vi "MultiCamExample.vi"() -> ()   [LabVIEW 2015]
panel:
  out "Numeric":i32
  out "Initialize Done":bool
  out "time":u32
  in  "Enabled/Disabled 1":bool
  in  "Load Picture 1":bool
  in  "Script Index 1":i32=1
  out "data string 1":string="1113.00\r\n935.00\r\n"
  out "VarName 1":string="up_ROI0_PM_Position_x\r\nup_ROI0_PM_Position_y\r\n"
  in  "Cam Index 1":i32=1
  in  "coordinate space 1":bool
  out "VarName 0":string="up_ROI0_PM_Position_x\r\nup_ROI0_PM_Position_y\r\n"
  in  "Script Index 0":i32
  in  "CameraName":string[](array[string])=["cam0"]
  in  "Load File Path":string[](array[string])=["C:\\Code\\Washers.png"]
  in  "script path":string[](array[string])=["C:\\Code\\iVision_20160509_Caliper_Coor -Cal\\Data\\Calibration"]
  in  "Cam Index 0":i32
  in  "Load Picture 0":bool
  in  "coordinate space 0":bool
  in  "Run":bool
  in  "Enabled/Disabled 0":bool
  in  "stop":bool
  out "data string 0":string="1113.00\r\n935.00\r\n"
  # "<- Run之前要改"
  # "<- Run之前要改"
  # "<- Run之前要改"
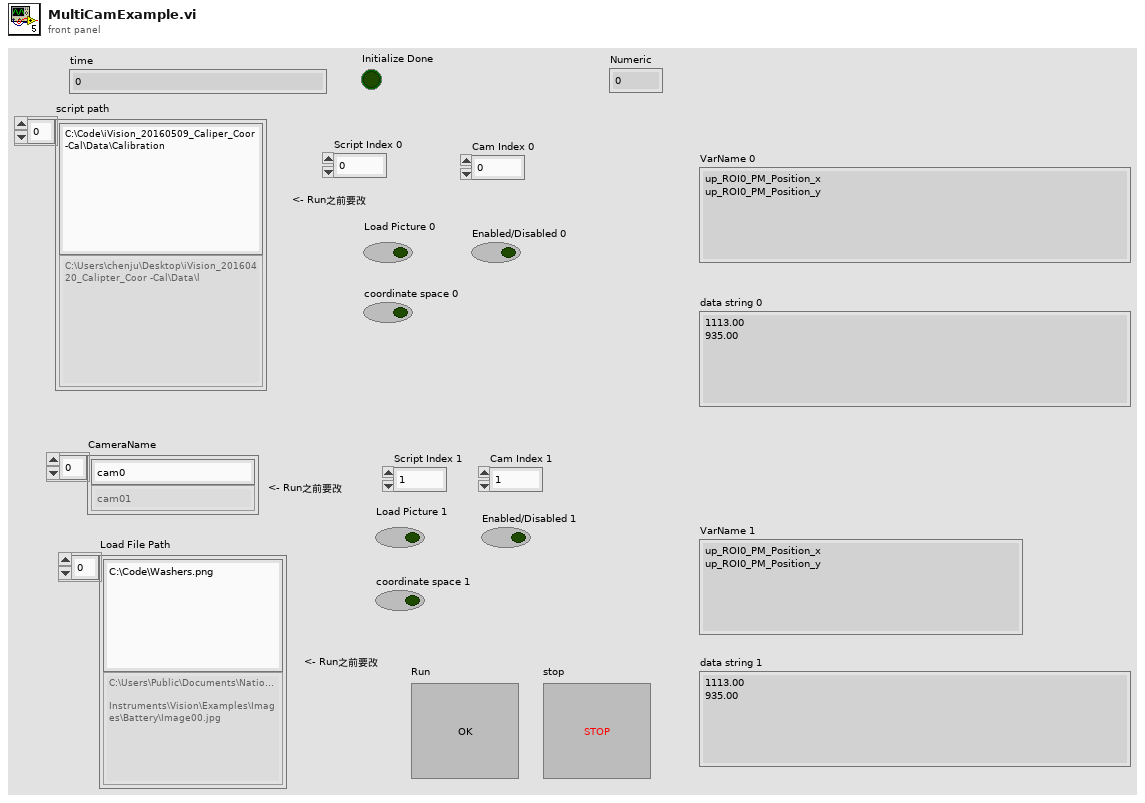
[diagram p1: front panel]
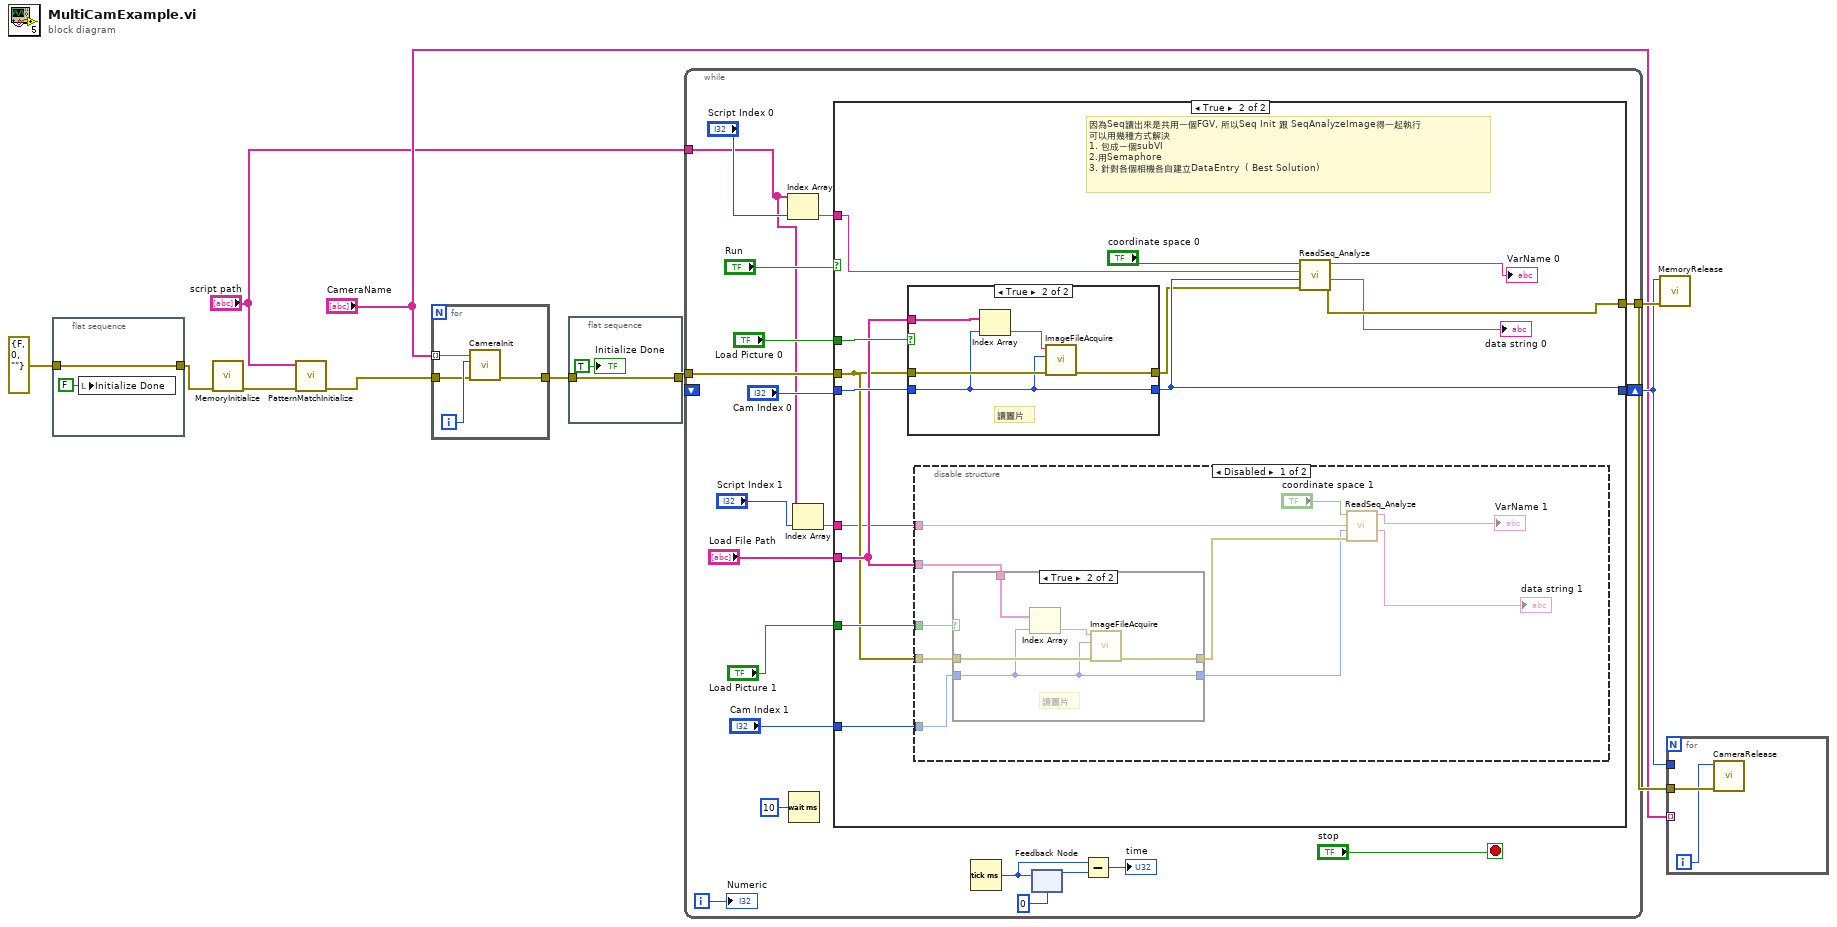
[diagram p0: block diagram]
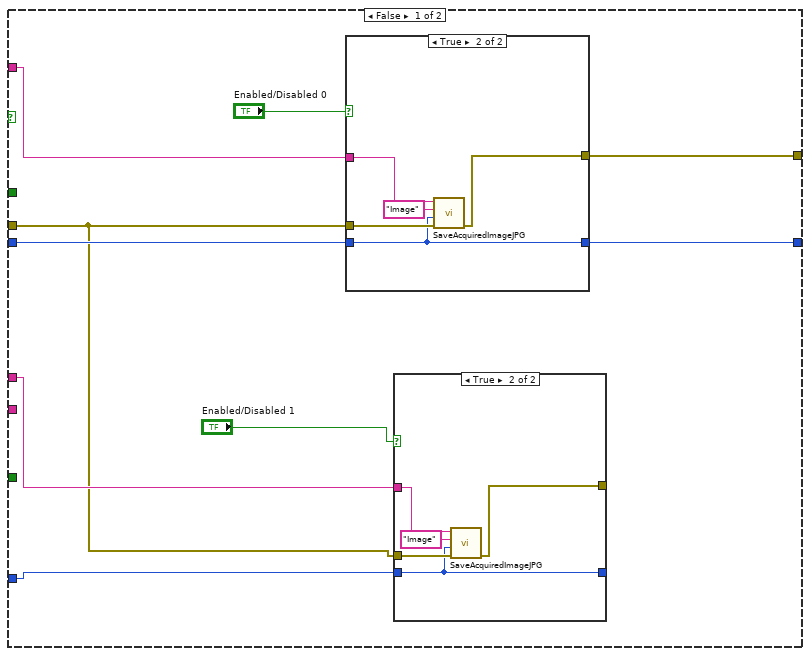
[diagram p2: hidden frame]
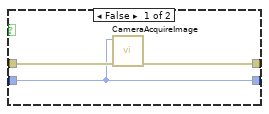
[diagram p5: hidden frame]
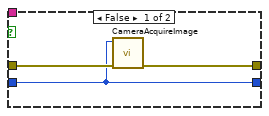
[diagram p7: hidden frame]
diagram:
  n1 = flat-sequence {
    tunnel: [w11] -> w2
    tunnel: errorcluster {"status"=FALSE, "code"=0, "source"=""} ("error in (no error)") -> [w11]
    frame #0 {
      n2 = local write "Initialize Done"(FALSE ("Initialize Done")) -> ()
    }
  }
  n3 = call "MemoryInitialize.vi"("error in (no error)"=w2) -> ("error out"=w7:errorcluster)  [unwired: 10 in]
  n4 = call "PatternMatchInitialize.vi"("Error In"=w7, "script path"="script path") -> ("Error Out"=w6:errorcluster)  [unwired: 9 in]
  n5 = for {
    tunnel: [w16] -> w3
    tunnel: "CameraName" -> [w15] mode=indexing
    tunnel: w6 -> [w13]
    i -> [w14]
    n6 = call "CameraInit.vi"("error in"=w13, "Index"=w14, "CameraName"=w15) -> ("error out"=w16:errorcluster)  [unwired: 7 in, 1 out]
  }
  n7 = flat-sequence {
    tunnel: [w18] -> w4
    tunnel: w3 -> [w18]
    frame #0 {
      "Initialize Done" <- TRUE ("Initialize Done")
    }
  }
  n8 = while {
    tunnel: w4 -> [w38]
    tunnel: [w37] -> w10
    shift-right: [w35] -> w9
    shift-left: _ -> [_]
    tunnel: "script path" -> [w20]
    i -> [w19]
    stop <- "stop" stop-if-true
    n9 = Index Array(array=w20, index="Script Index 0") -> (element=w32:string)
    n10 = Wait (ms)(milliseconds to wait=u32 10) -> ()  [unwired: 1 out]
    n11 = Index Array(array=w20, index="Script Index 1") -> (element=w27:string)
    n12 = case shown="True" "Run" {
      tunnel: w38 -> [w41 w68]
      tunnel: [w47 w76] -> w37
      tunnel: "Load Picture 0" -> [_ w75]
      tunnel: "Cam Index 0" -> [w46 w74]
      tunnel: [w45 w73] -> w35
      tunnel: w32 -> [w44 w72]
      tunnel: "Load File Path" -> [_ w71]
      tunnel: "Load Picture 1" -> [_ w70]
      tunnel: "Cam Index 1" -> [w40 w69]
      tunnel: w27 -> [w42 w67]
      frame False {
        n13 = case shown="True" "Enabled/Disabled 0" {
          tunnel: w41 -> [w57 w62]
          tunnel: [w57 w61] -> w47
          tunnel: w44 -> [_ w60]
          tunnel: w46 -> [w56 w58]
          tunnel: [w56 w58] -> w45
          frame False {
          }
          frame True {
            n14 = call "SaveAcquiredImageJPG.vi"("error in"=w62, "Index"=w58, "File Name"="Image", "Folder Path"=w60) -> ("error out"=w61:errorcluster)  [unwired: 4 in, 3 out]
          }
        }
        n15 = case shown="True" "Enabled/Disabled 1" {
          tunnel: w41 -> [w50 w55]
          tunnel: [w50 w54] -> _
          tunnel: w42 -> [_ w53]
          tunnel: w40 -> [w49 w51]
          tunnel: [w49 w51] -> _
          frame False {
          }
          frame True {
            n16 = call "SaveAcquiredImageJPG.vi"("error in"=w55, "Index"=w51, "File Name"="Image", "Folder Path"=w53) -> ("error out"=w54:errorcluster)  [unwired: 4 in, 3 out]
          }
        }
      }
      frame True {
        # "因為Seq讀出來是共用一個FGV, 所以Seq Init 跟 SeqAnalyzeImage得一起執行\n可以用幾種方式解決\n1. 包成一個subVI\n2.用Semaphore\n3. 針對各個相機各自建立DataEntry  ( Best Solution)"
        n17 = case shown="True" w75 {
          tunnel: w68 -> [w97 w102]
          tunnel: [w96 w101] -> w66
          tunnel: w74 -> [w95 w100]
          tunnel: [w95 w100] -> w73
          tunnel: w71 -> [_ w98]
          frame False {
            n18 = call "CameraAcquireImage.vi"("error in"=w97, "Index"=w95) -> ("error out"=w96:errorcluster)  [unwired: 8 in, 1 out]
          }
          frame True {
            # "讀圖片"
            n19 = Index Array(array=w98, index=w100) -> (element=w99:string)
            n20 = call "ImageFileAcquire.vi"("error in"=w102, "Index"=w100, "File Path"=w99) -> ("error out"=w101:errorcluster)  [unwired: 7 in, 1 out]
          }
        }
        n21 = disable-structure shown="Disabled" {
          disable-tunnel: w71 -> [w86 _]
          disable-tunnel: w70 -> [w85 _]
          disable-tunnel: w69 -> [w84 _]
          disable-tunnel: w68 -> [w83 _]
          disable-tunnel: w67 -> [w82 _]
          frame Disabled {
            n22 = case shown="True" w85 {
              tunnel: w83 -> [w89 w94]
              tunnel: [w88 w93] -> w78
              tunnel: w84 -> [w87 w92]
              tunnel: [w87 w92] -> w77
              tunnel: w86 -> [_ w90]
              frame False {
                n23 = call "CameraAcquireImage.vi"("error in"=w89, "Index"=w87) -> ("error out"=w88:errorcluster)  [unwired: 8 in, 1 out]
              }
              frame True {
                # "讀圖片"
                n24 = Index Array(array=w90, index=w92) -> (element=w91:string)
                n25 = call "ImageFileAcquire.vi"("error in"=w94, "Index"=w92, "File Path"=w91) -> ("error out"=w93:errorcluster)  [unwired: 7 in, 1 out]
              }
            }
            n26 = call "ReadSeq_Analyze.vi"("error in (no error)"=w78, "Cam Index"=w77, "script path"=w82, "coordinate space"="coordinate space 1") -> ("data string"=→"data string 1":string, "VarName"=→"VarName 1":string)  [unwired: 4 in, 2 out]
          }
          frame Enabled {
          }
        }
        n27 = call "ReadSeq_Analyze.vi"("error in (no error)"=w66, "Cam Index"=w73, "script path"=w72, "coordinate space"="coordinate space 0") -> ("error out"=w76:errorcluster, "data string"=→"data string 0":string, "VarName"=→"VarName 0":string)  [unwired: 4 in, 1 out]
      }
    }
    n28 = Tick Count (ms)() -> (millisecond timer value=w23:u32)
    n29 = feedback #1(u32 0 ("millisecond timer value")) -> (w24:u32)
    n30 = feedback-in #1(w23) -> ()
    n31 = Subtract(x=w23, y=w24) -> (x-y=→"time":u32)
    "Numeric" <- w19
  }
  n32 = call "MemoryRelease.vi"("error in"=w10, "Index"=w9) -> ()  [unwired: 8 in, 2 out]
  n33 = for {
    tunnel: w10 -> [w104]
    tunnel: w9 -> [_]
    tunnel: "CameraName" -> [_] mode=indexing
    i -> [w103]
    n34 = call "CameraRelease.vi"("error in"=w104, "Index"=w103) -> ()  [unwired: 8 in, 2 out]
  }
